vi "GotoJog.vi"(0 "reference":refnum<visa-resource-name>, 5 "Position Y":i32=100 min=1 max=500000, 7 "Position X":i32=100 min=1 max=500000, 9 "Position Z":i32=100 min=1 max=500000, 11 "Position F":i32=100 min=1 max=500000) -> (4 "reference dup":refnum<visa-resource-name>, 8 "OK Done":bool, 15 "error OUT":errorcluster)   [LabVIEW 2019]
panel:
  # "Port Number 0=COM1"
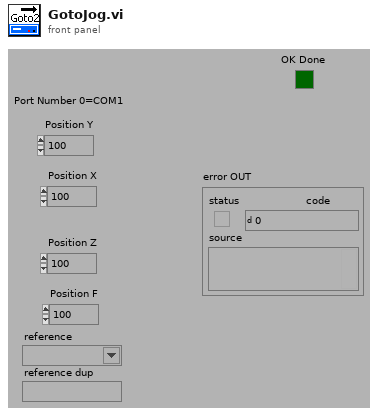
[diagram p1: front panel]
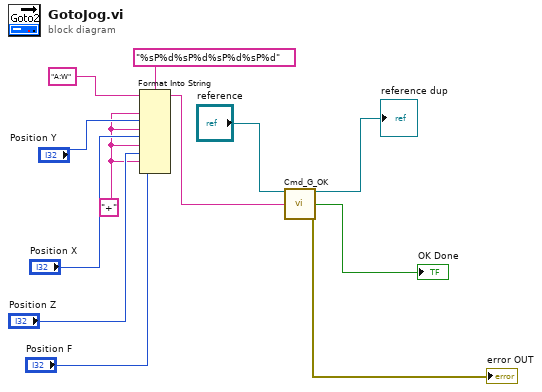
[diagram p0: block diagram]
diagram:
  w4 = "+"
  n1 = Format Into String(format string="%sP%d%sP%d%sP%d%sP%d", initial string="A:W", w4, "Position Y", w4, "Position X", w4, "Position Z", w4, "Position F") -> (resulting string=w10:string)  [unwired: 1 in, 1 out]
  n2 = call "Cmd_G_OK.vi"("reference"="reference", "Command String"=w10) -> ("reference dup"=→"reference dup":refnum<visa-resource-name>, "OK Done"=→"OK Done":bool, "error OUT"=→"error OUT":errorcluster)  [unwired: 11 in]
